vi "Test Log Update Table.vi"(8 "error in (no error)":errorcluster, 11 "Test Info in":refnum<class "Test Info.lvclass">) -> (0 "error out":errorcluster, 3 "Test Info out":refnum<class "Test Info.lvclass">)   [LabVIEW 2023, in "Data Analysis.lvlib" / "Test Info.lvlib" / "Test Info.lvclass"]
uses:
  Test Info.lvclass
  Test Info.lvclass/Test Info.ctl
  Data Analysis.lvlib
  HardwareAbstractionLayer_LVOOP/Database/Database.lvclass
  <vilib>/Utility/miscctls.llb/LVRowAndColumnUnsignedTypeDef.ctl
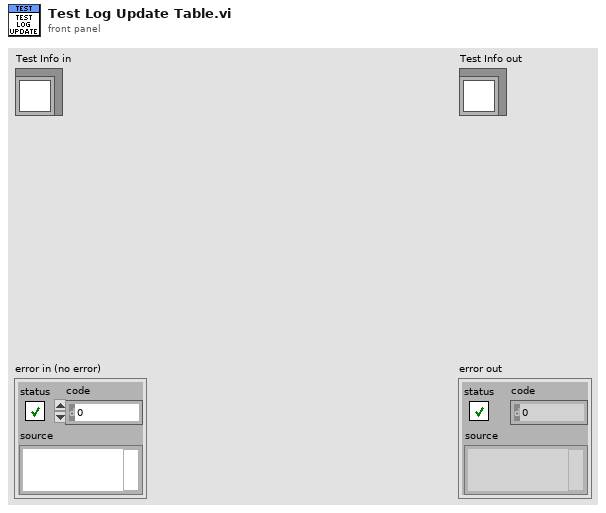
[diagram p1: front panel]
types:
  T1 = typedef "LVRowAndColumnUnsignedTypeDef.ctl" = cluster{"Row":u32, "Column":u32}
  T2 = cluster{"table":string, "condition":string, "columns":string[]}
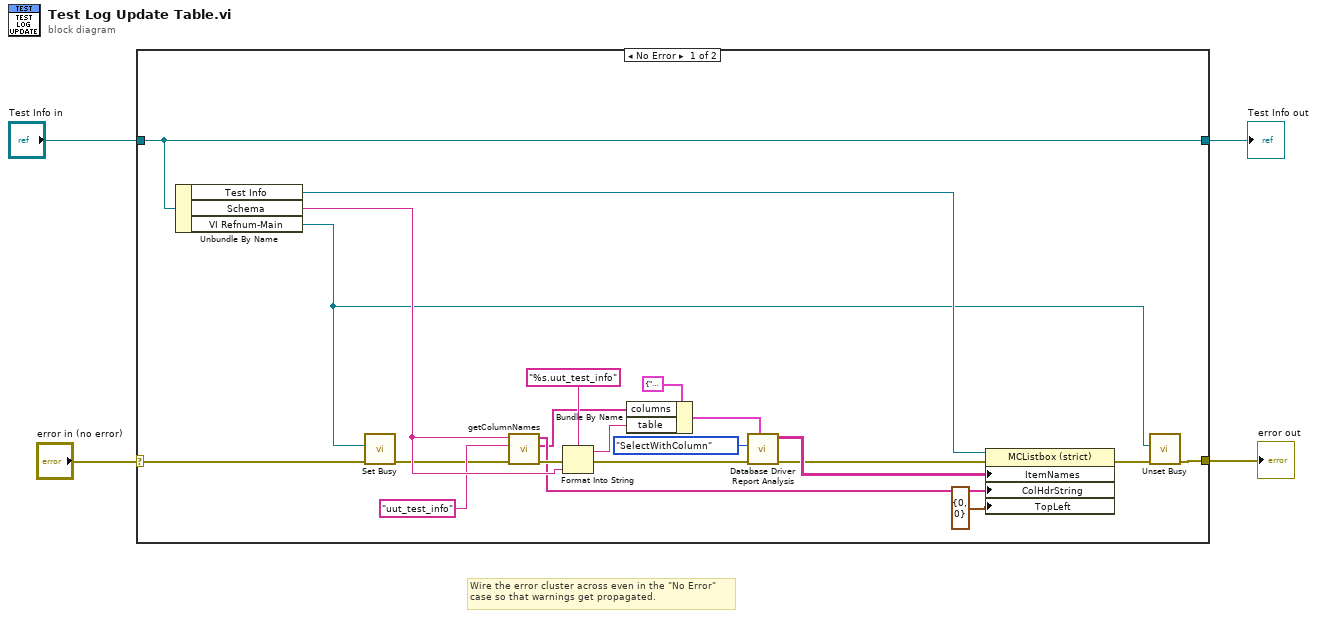
[diagram p0: block diagram]
diagram:
  # "Wire the error cluster across even in the \"No Error\"\ncase so that warnings get propagated."
  n1 = case shown="No Error" "error in (no error)" {
    selector: "error in (no error)" -> [w10 w27]
    tunnel: [w7 w27] -> w3
    tunnel: [w25 w26] -> w1
    tunnel: "Test Info in" -> [w25 w26]
    frame No Error {
      n2 = Unbundle By Name(w25) -> ("Test Info"=w24:refnum<vi>, "Schema"=w23:string, "VI Refnum-Main"=w6:refnum<vi>)
      n3 = call <vilib>:"Set Busy.vi"("error in (no error)"=w10, "VI reference (current VI)"=w6) -> ("error out"=w9:errorcluster)  [unwired: 8 in, 1 out]
      n4 = call "getColumnNames.vi"("error in (no error)"=w9, "tableName"="uut_test_info" ("schema"), "schema"=w23) -> ("error out"=w21:errorcluster, "columnNamesForQuery"=w11:string[], "columnNames"=w12:string[])  [unwired: 6 in]
      n5 = Format Into String(format string="%s.uut_test_info" ("schema"), error in=w21, w23) -> (resulting string=w15:string, error out=w17:errorcluster)  [unwired: 1 in]
      n6 = Bundle By Name(cluster=T2 {"table"="", "condition"="", "columns"=[]} ("SQLTableData"), "columns"=w11, "table"=w15) -> (w14:T2)
      n7 = call "Database Driver Report Analysis.vi"("SQLTableData"=w14, "error in"=w17, "Select"=enum16{"SelectWithQuery", "SelectWithColumn"}."SelectWithColumn") -> ("error out"=w18:errorcluster, "data"=w19:string[][])  [unwired: 5 in, 2 out]
      n8 = property class="MCListbox (strict)"(reference=w24, error in=w18, "ItemNames"=w19, "ColHdrString"=w12, "TopLeft"=T1 {"Row"=0, "Column"=0} ("Top Left Visible Cell")) -> (error out=w8:errorcluster)  [unwired: 1 out]
      n9 = call <vilib>:"Unset Busy.vi"("error in (no error)"=w8, "VI reference (current VI)"=w6) -> ("error out"=w7:errorcluster)  [unwired: 9 in]
    }
    frame Error {
    }
  }
  "error out" <- w3
  "Test Info out" <- w1
